vi "Actor Core.vi"(8 "error in":errorcluster, 11 "Nested in":refnum<class "Root Actor.lvclass">) -> (0 "error out":errorcluster, 3 "Actor out":refnum<class "Actor.lvclass">)   [LabVIEW 2024, in "Root Actor.lvlib" / "Root Actor.lvclass"]
doc: "(<B>Filename</B>: Actor Framework.lvlib:Actor.lvclass:Actor Core.vi)\n\nReceives messages to the actor, reacts to them, and initiates any error handling that may shut the actor down.\n\nDescendant classes may override this VI to append parallel tasks for the actor to complete while it handles messages. Overrides use the Call Parent Method node."
uses:
  Root Actor.lvclass
  C:/Program Files/National Instruments/LabVIEW 2024/vi.lib/ActorFramework/Actor/Actor.lvclass
  <vilib>/ActorFramework/Actor/Actor.lvclass
  Chef States/INIT/INIT.lvclass
  <vilib>/ActorFramework/Actor/Actor.lvclass/Actor.ctl
  <vilib>/ActorFramework/Message Enqueuer/Message Enqueuer.lvclass/Message Enqueuer.ctl
  Root Actor.lvclass/Root Actor.ctl
  <vilib>/ActorFramework/Message Enqueuer/Init from Existing Queue.vi
  <vilib>/ActorFramework/Message Enqueuer/Enqueue.vi
  <vilib>/ActorFramework/Stop Msg/Stop Msg.lvclass
  C:/Program Files/National Instruments/LabVIEW 2024/vi.lib/ActorFramework/Message/Message.lvclass
  <vilib>/ActorFramework/Message Priority Queue/Priority Enqueue.vi
  <vilib>/ActorFramework/Message Enqueuer/Message Enqueuer.lvclass
panel:
  out "State String":string
  in  "Exit Button":bool
  in  "Start Button":bool
  # "Current State"
  # "Made by Ramazan Burak Korkmaz- 2024"
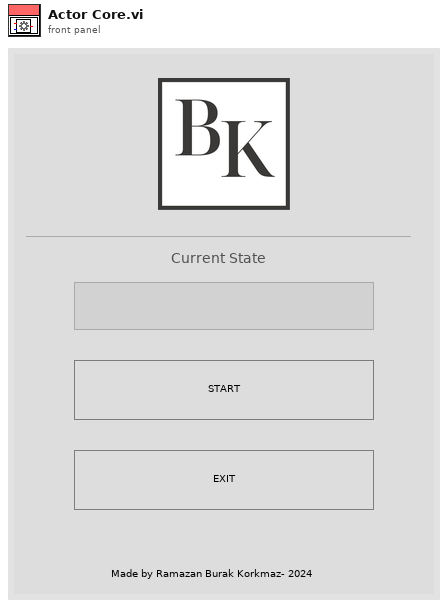
[diagram p1: front panel]
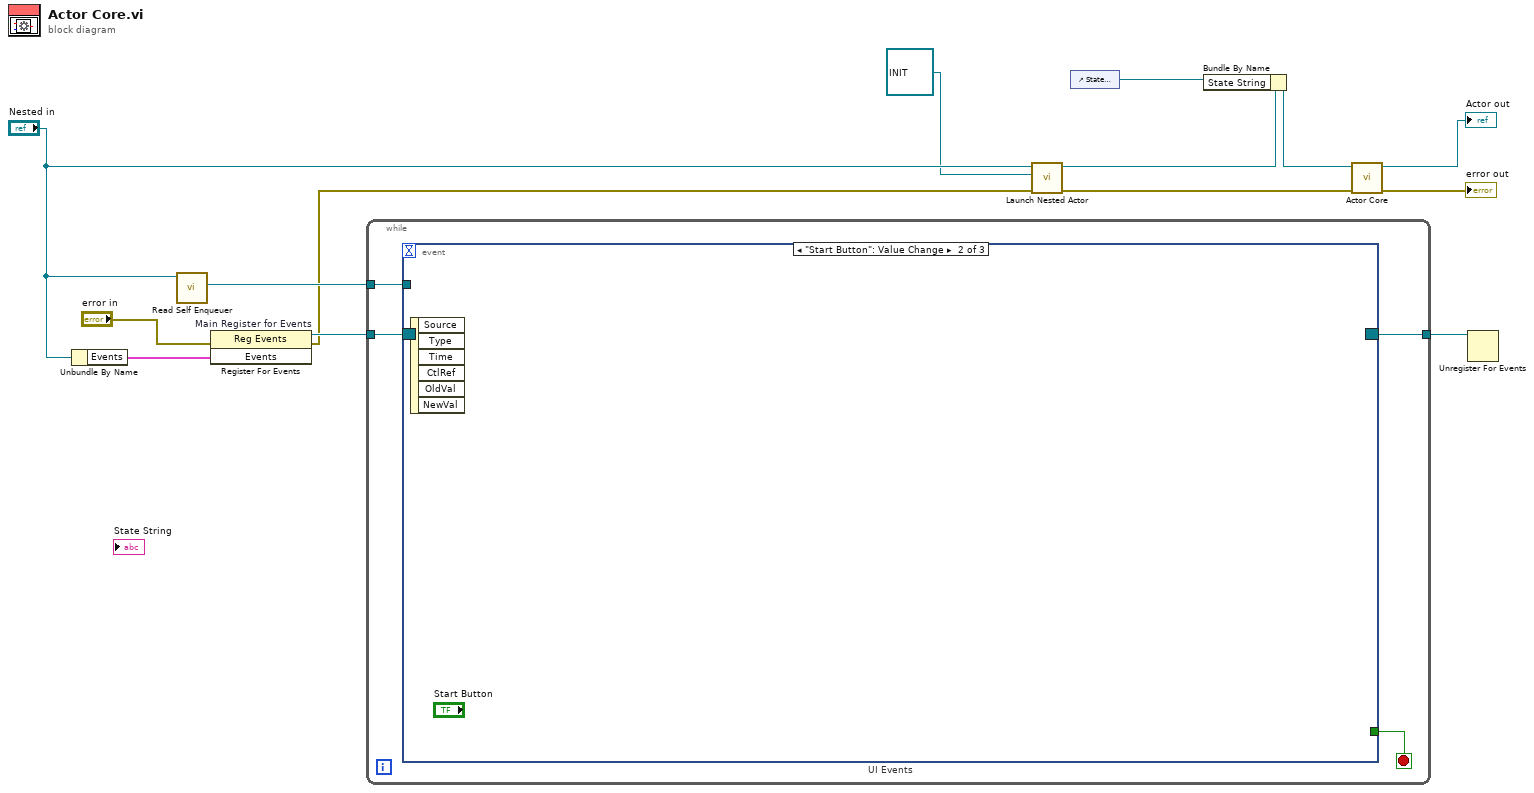
[diagram p0: block diagram]
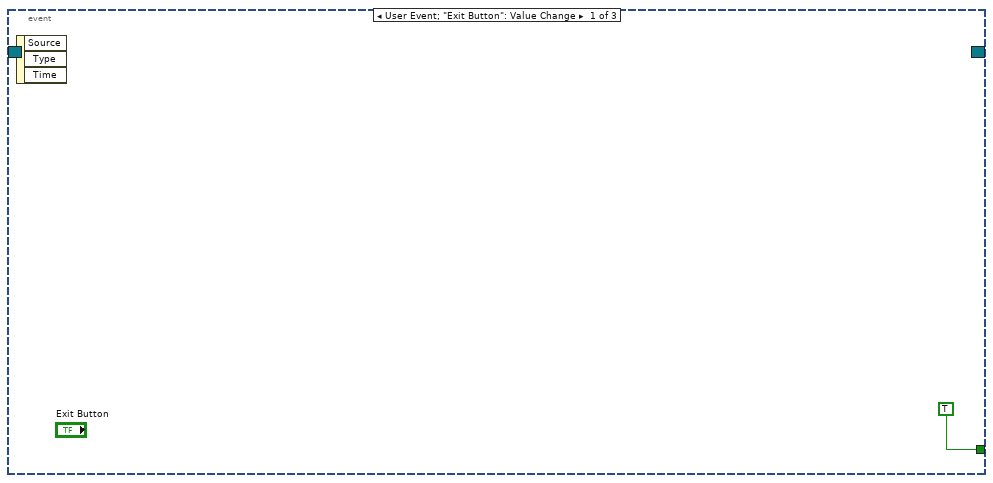
[diagram p2: hidden frame]
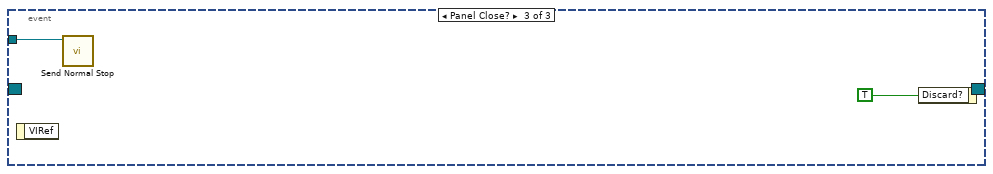
[diagram p3: hidden frame]
diagram:
  n1 = Unbundle By Name("Nested in") -> ("Events"=w11:cluster{"Stop":refnum<user-event>})
  n2 = call <vilib>:"Read Self Enqueuer.vi"("Actor"="Nested in") -> ("Self Enqueuer"=w9:refnum<class "Message Enqueuer.lvclass">)  [unwired: 10 in]
  n3 = register-events "Main Register for Events"(error in="error in", w11) -> (reference out=w12:refnum<event-registration>, error out=w7:errorcluster)  [unwired: 1 in]
  n4 = while {
    tunnel: w12 -> [w18]
    tunnel: [w16] -> w10
    tunnel: w9 -> [w15]
    stop <- w17 stop-if-true
    n5 = event "UI Events" shown="[1] \"Start Button\": Value Change" {
      selector: w18 -> [_ _ _]
      dyn-events: [_ _ _] -> w16
      timeout: _ -> [_ _ _]
      tunnel: [TRUE _ _] -> w17
      tunnel: w15 -> [_ _ w20]
      event User Event; "Exit Button": Value Change {
        n6 = event-data() -> ()  [unwired: 1 in, 3 out]
      }
      event "Start Button": Value Change {
        n7 = event-data() -> ()  [unwired: 1 in, 6 out]
      }
      event Panel Close? {
        n8 = event-data() -> ()  [unwired: 1 in, 1 out]
        n9 = call <vilib>:"Send Normal Stop.vi"("Message Enqueuer"=w20) -> ()  [unwired: 10 in, 1 out]
        n10 = event-data("Discard?"=TRUE) -> ()  [unwired: 1 in, 1 out]
      }
    }
  }
  n11 = call <vilib>:"Launch Nested Actor.vi"("error in (no error)"=w7, "Nested Actor"=refnum<class "INIT.lvclass"> refnum ("Chef States.lvlib:INIT.lvclass"), "Caller Actor in"="Nested in") -> ("error out"=w4:errorcluster, "Caller Actor out"=w5:refnum<class "Root Actor.lvclass">)  [unwired: 6 in, 1 out]
  n12 = control-ref of="State String"() -> (w1:refnum<vi>)
  n13 = Bundle By Name(cluster=w5, "State String"=w1) -> (w2:refnum<class "Root Actor.lvclass">)
  n14 = call-parent "Actor Core.vi"("error in"=w4, "Actor in"=w2) -> ("error out"=→"error out":errorcluster, "Actor out"=→"Actor out":refnum<class "Actor.lvclass">)  [unwired: 8 in]
  n15 = Unregister For Events(event registration refnum=w10) -> ()  [unwired: 1 in, 1 out]
